vi "Disconnect.vi"(8 "error in (no error)":errorcluster, 11 "PicoScope 3000a in":refnum<class "PicoScope 3000a.lvclass">) -> (0 "error out":errorcluster, 3 "PicoScope 3000a out":refnum<class "PicoScope 3000a.lvclass">)   [LabVIEW 2018, in "PicoScope 3000a.lvlib" / "PicoScope 3000a.lvclass"]
doc: "This Override method is used finalize the communication session with the Oscope instrument."
uses:
  PicoScope 3000a.lvclass
  PicoScope 3000a.lvclass/PicoScope 3000a.ctl
  <instrlib>/PicoScope/PicoScope.lvlib
  ps3000a.dll
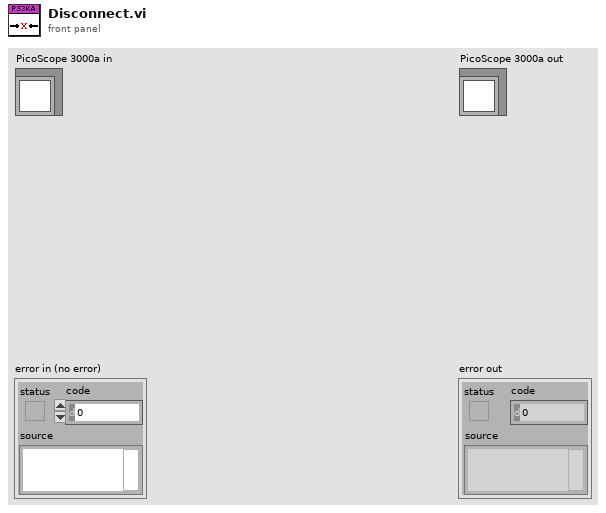
[diagram p1: front panel]
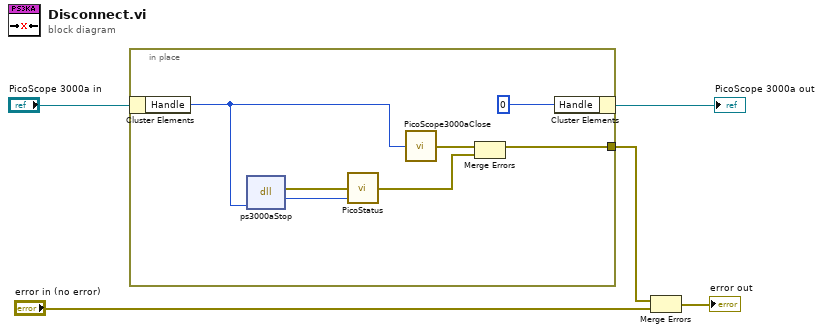
[diagram p0: block diagram]
diagram:
  n1 = in-place {
    in-place-border: [w6] -> w2
    n2 = in-place-cluster #1("PicoScope 3000a in") -> ("Handle"=w11:i16)
    n3 = dll-call lib="ps3000a.dll" fn="ps3000aStop" label="ps3000.dll:_ps3000_stop"("handle"=w11) -> (error out=w10:errorcluster, "PICO_STATUS"=w9:u32)  [unwired: 4 in, 1 out]
    n4 = call <instrlib>:"PicoStatus.vi"("PICO STATUS"=w9, "error in"=w10) -> ("error out"=w8:errorcluster)  [unwired: 1 in]
    n5 = call <instrlib>:"PicoScope3000aClose.vi"("handle"=w11) -> ("error out"=w7:errorcluster)
    n6 = Merge Errors(w7, w8) -> (w6:errorcluster)
    n7 = in-place-cluster #1("Handle"=i16 0) -> (→"PicoScope 3000a out":refnum<class "PicoScope 3000a.lvclass">)
  }
  n8 = Merge Errors(w2, "error in (no error)") -> (→"error out":errorcluster)
